vi "MovingAverage.vi"() -> ()   [LabVIEW 2014]
panel:
  out "Numeric 2":i32
  in  "Numeric":i32
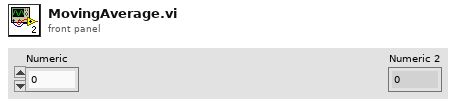
[diagram p1: front panel]
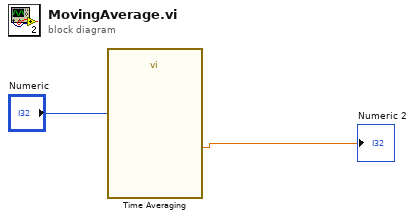
[diagram p0: block diagram]
diagram:
  n1 = call "Time Averaging"("input signal"="Numeric") -> ("time avg. signal"=→"Numeric 2":dbl)  [unwired: 15 in, 3 out]
